vi "Get.vi"(8 "error in (no error)":errorcluster, 11 "AbstractBattery in":refnum<class "AbstractBattery.lvclass">) -> (0 "error out":errorcluster, 2 "Output":dbl, 3 "AbstractBattery out":refnum<class "AbstractBattery.lvclass">)   [LabVIEW 2011, in "AbstractBattery.lvclass"]
uses:
  AbstractBattery.lvclass
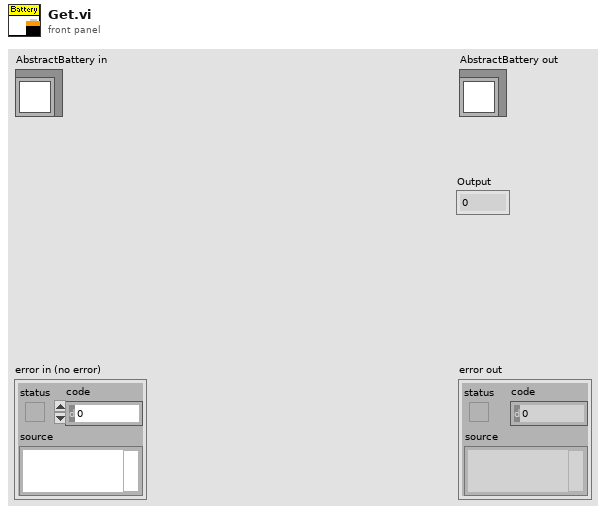
[diagram p1: front panel]
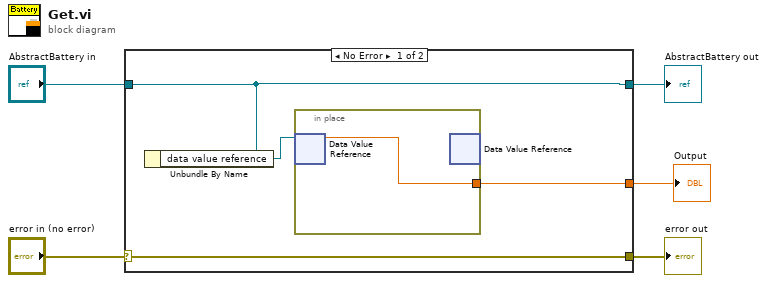
[diagram p0: block diagram]
diagram:
  n1 = case shown="No Error" "error in (no error)" {
    selector: "error in (no error)" -> [w9 w11]
    tunnel: [w9 w11] -> w4
    tunnel: [w7 w12] -> w2
    tunnel: "AbstractBattery in" -> [w7 w12]
    tunnel: [w6 _] -> w1
    frame No Error {
      n2 = Unbundle By Name(w7) -> ("data value reference"=w8:refnum<data-value>)
      n3 = in-place {
        in-place-border: [w10] -> w6
        n4 = in-place-dvr #1(w8) -> (w10:dbl)  [unwired: 1 out]
        n5 = in-place-dvr #1() -> ()  [unwired: 1 in, 2 out]
      }
    }
    frame Error {
    }
  }
  "error out" <- w4
  "AbstractBattery out" <- w2
  "Output" <- w1
